vi "SwerveJoystickStrafeScaling.vi"(0 "Raw Joystick X":dbl, 5 "Raw Joystick Y":dbl, 7 "Auto Control":bool, 9 "Strafe Deadband":dbl(slide)=0.05 min=0.0 max=0.4 scale=0.0..0.4, 11 "Strafe Scaling":dbl(slide)=2.0 min=1.0 max=4.0 scale=1.0..4.0) -> (4 "In Deadband":bool, 8 "Scaled Joystick X":dbl, 15 "Scaled Joystick Y":dbl)   [LabVIEW 2019]
doc: "Applies a deadband and nonlinear scaling to the strafe axes of a swerve drive. Includes a hook to override the non-linear deadband and scaling when the rotation is under autonomous control. Includes a de-saturation check to handle compounding drive commands from different controllers (e.g. direct driver control + auto targeting)."
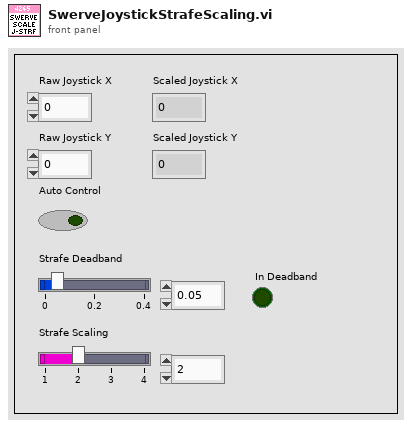
[diagram p1: front panel]
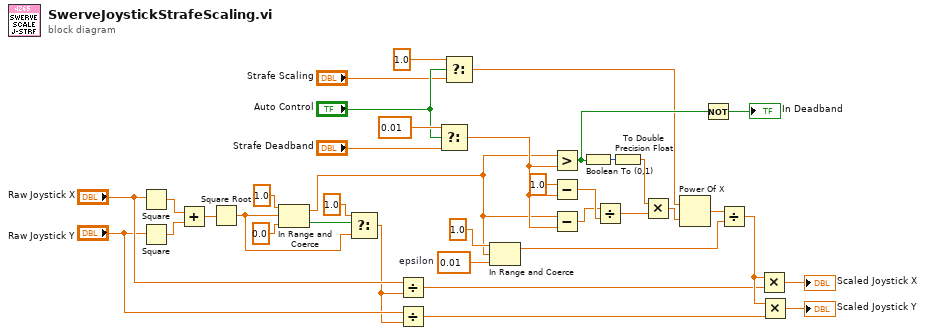
[diagram p0: block diagram]
diagram:
  w30 = 0.01  # epsilon
  n1 = Square(x="Raw Joystick X") -> (x^2=w27:dbl)
  n2 = Square(x="Raw Joystick Y") -> (x^2=w26:dbl)
  n3 = Add(x=w27, y=w26) -> (x+y=w28:dbl)
  n4 = Square Root(x=w28) -> (sqrt(x)=w7:dbl)
  n5 = In Range and Coerce(upper limit=1.0, x=w7, lower limit=0.0 ("upper limit")) -> (coerced(x)=w1:dbl, In Range?=w9:bool)
  n6 = Select(t=1.0, s=w9, f=w7) -> (s? t:f=w2:dbl)
  n7 = Divide(x="Raw Joystick X", y=w2) -> (x/y=w6:dbl)
  n8 = Divide(x="Raw Joystick Y", y=w2) -> (x/y=w3:dbl)
  n9 = Select(t=0.01, s="Auto Control", f="Strafe Deadband") -> (s? t:f=w12:dbl)
  n10 = Select(t=1.0, s="Auto Control", f="Strafe Scaling") -> (s? t:f=w13:dbl)
  n11 = In Range and Coerce(upper limit=1.0, x=w1, lower limit=w30) -> (coerced(x)=w29:dbl)  [unwired: 1 out]
  n12 = Greater?(x=w1, y=w12) -> (0:w35:bool)
  n13 = Subtract(x=1.0, y=w12) -> (x-y=w24:dbl)
  n14 = Subtract(x=w1, y=w12) -> (x-y=w22:dbl)
  n15 = Boolean To (0,1)(Boolean=w35) -> (0, 1=w20:i16)
  n16 = Divide(x=w22, y=w24) -> (x/y=w25:dbl)
  n17 = To Double Precision Float(number=w20) -> (double precision float=w21:dbl)
  n18 = Multiply(x=w21, y=w25) -> (x*y=w36:dbl)
  n19 = Power Of X(1:w36, 2:w13) -> (0:w37:dbl)
  n20 = Not(x=w35) -> (.not. x?=→"In Deadband":bool)
  n21 = Divide(x=w37, y=w29) -> (x/y=w32:dbl)
  n22 = Multiply(x=w32, y=w6) -> (x*y=→"Scaled Joystick X":dbl)
  n23 = Multiply(x=w32, y=w3) -> (x*y=→"Scaled Joystick Y":dbl)
